vi "SpinCoaterArray2String_v04.vi"(3 "Time Start":dbl[unit], 4 "Program Spin Coater\nSpeed (rpm)          Time (s)":dbl[][](array[numeric])) -> (0 "Prg Spin Coater small":dbl[][](array[numeric]), 1 "remote control String":string)   [LabVIEW 2020, in "SpinCoater.lvclass"]
uses:
  <instrlib>/Classes/SpinCoater/SpinCoater.lvclass
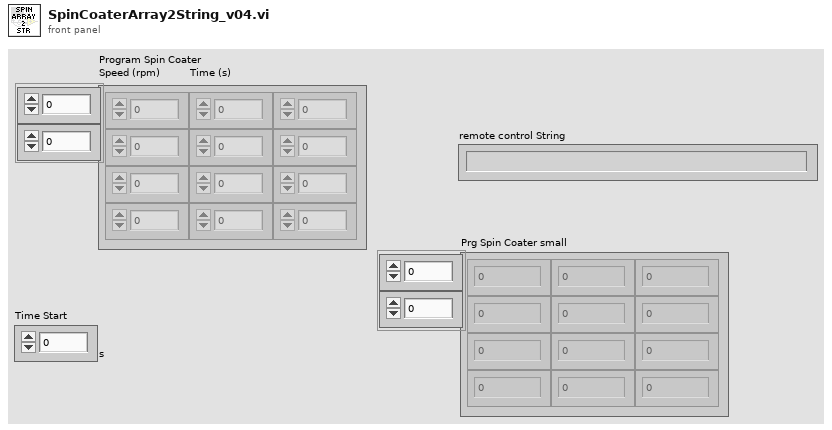
[diagram p1: front panel]
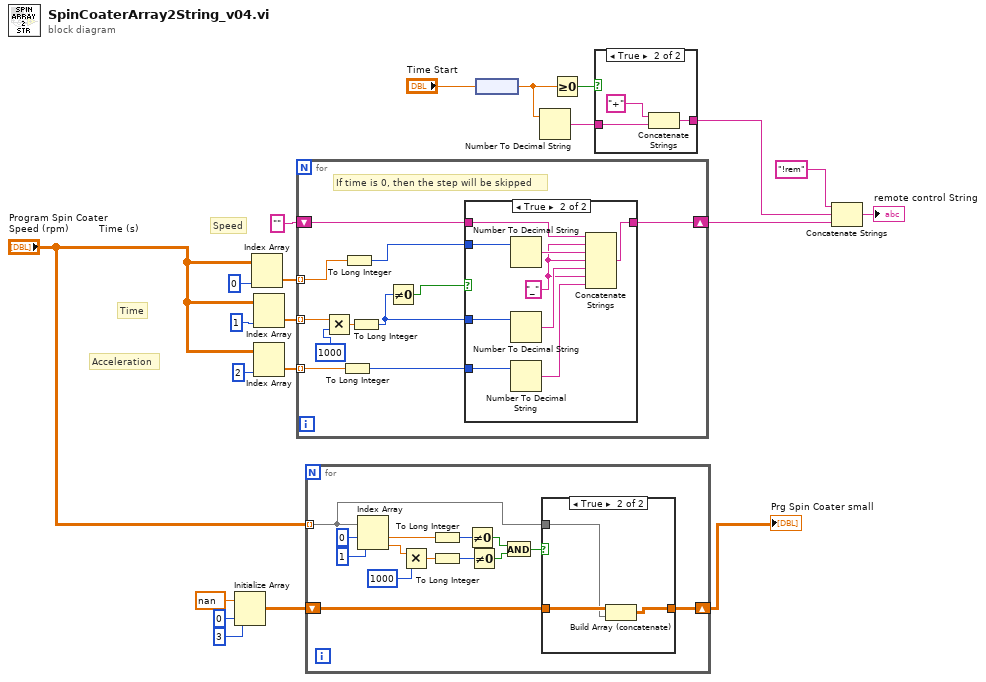
[diagram p0: block diagram]
diagram:
  # "Acceleration"
  # "Time"
  # "Speed"
  n1 = Initialize Array(nan ("element"), 0 ("dimension size"), 3 ("dimension size")) -> (w2:dbl[][])
  n2 = Index Array(array="Program Spin Coater\nSpeed (rpm)          Time (s)", index (col)=0 ("disabled index (col)")) -> (element=w19:dbl[])  [unwired: 1 in]
  n3 = Index Array(array="Program Spin Coater\nSpeed (rpm)          Time (s)", index (col)=1 ("disabled index (col)")) -> (element=w18:dbl[])  [unwired: 1 in]
  n4 = Index Array(array="Program Spin Coater\nSpeed (rpm)          Time (s)", index (col)=2 ("disabled index (col)")) -> (element=w7:dbl[])  [unwired: 1 in]
  n5 = for {
    tunnel: w19 -> [w32] mode=indexing
    tunnel: w18 -> [w25] mode=indexing
    shift-right: [w29] -> w9
    shift-left: "" ("string") -> [w30]
    tunnel: w7 -> [w28] mode=indexing
    # "If time is 0, then the step will be skipped"
    n6 = Multiply(x=w25, y=1000) -> (x*y=w26:dbl)
    n7 = To Long Integer(number=w28) -> (32bit integer=w27:i32)
    n8 = To Long Integer(number=w32) -> (32bit integer=w31:i32)
    n9 = To Long Integer(number=w26) -> (32bit integer=w23:i32)
    n10 = Not Equal To 0?(x=w23) -> (x != 0?=w22:bool)
    n11 = case shown="True" w22 {
      tunnel: w31 -> [_ w42]
      tunnel: w23 -> [_ w41]
      tunnel: w30 -> [w33 w38]
      tunnel: [w33 w37] -> w29
      tunnel: w27 -> [_ w36]
      frame False {
      }
      frame True {
        w35 = "_" ("string")
        n12 = Number To Decimal String(number=w42) -> (decimal integer string=w40:string)  [unwired: 1 in]
        n13 = Number To Decimal String(number=w41) -> (decimal integer string=w39:string)  [unwired: 1 in]
        n14 = Number To Decimal String(number=w36) -> (decimal integer string=w34:string)  [unwired: 1 in]
        n15 = Concatenate Strings(w38, w35, w40, w35, w39, w35, w34) -> (w37:string)
      }
    }
  }
  n16 = for {
    tunnel: "Program Spin Coater\nSpeed (rpm)          Time (s)" -> [w48] mode=indexing
    shift-right: [w46] -> w1
    shift-left: w2 -> [w47]
    n17 = Index Array(array=w48, index #1=0 ("index"), index #2=1 ("index")) -> (element #1=w54:dbl, element #2=w44:dbl)
    n18 = Multiply(x=w44, y=1000) -> (x*y=w45:dbl)
    n19 = To Long Integer(number=w54) -> (32bit integer=w50:i32)
    n20 = To Long Integer(number=w45) -> (32bit integer=w51:i32)
    n21 = Not Equal To 0?(x=w50) -> (x != 0?=w53:bool)
    n22 = Not Equal To 0?(x=w51) -> (x != 0?=w52:bool)
    n23 = And(x=w53, y=w52) -> (x .and. y?=w49:bool)
    n24 = case shown="True" w49 {
      tunnel: w48 -> [_ w59]
      tunnel: w47 -> [w57 w60]
      tunnel: [w57 w58] -> w46
      frame False {
      }
      frame True {
        n25 = Build Array (concatenate)(w60, w59) -> (w58:dbl[][])
      }
    }
  }
  "Prg Spin Coater small" <- w1
  n26 = node("Time Start") -> (w13:dbl)
  n27 = Number To Decimal String(number=w13) -> (decimal integer string=w12:string)  [unwired: 1 in]
  n28 = Greater Or Equal To 0?(x=w13) -> (x >= 0?=w14:bool)
  n29 = case shown="True" w14 {
    tunnel: w12 -> [w61 w63]
    tunnel: [w61 w62] -> w11
    frame False {
    }
    frame True {
      n30 = Concatenate Strings("+", w63) -> (w62:string)
    }
  }
  n31 = Concatenate Strings("!rem" ("string"), w11, w9) -> (→"remote control String":string)
